vi "printDaqSyncComponent.vi"(8 "error in":errorcluster, 9 "Indent":i32, 10 "TreeRef":refnum<vi>, 11 "baseObject in":refnum<class "IBaseObject.lvclass">) -> (0 "error out":errorcluster, 3 "baseObject out":refnum<class "IBaseObject.lvclass">)   [LabVIEW 2022 SP3, in "openDAQ.lvlib" / "daqUtils.lvlib" / "Tree.lvlib"]
uses:
  Tree.lvlib
  ISyncComponent/ISyncComponent.lvclass
  IBaseObject/IBaseObject.lvclass
  IBaseObject/Polymorphic/queryInterface/querySyncComponentInterface.vi
  IComponent/IComponent.lvclass
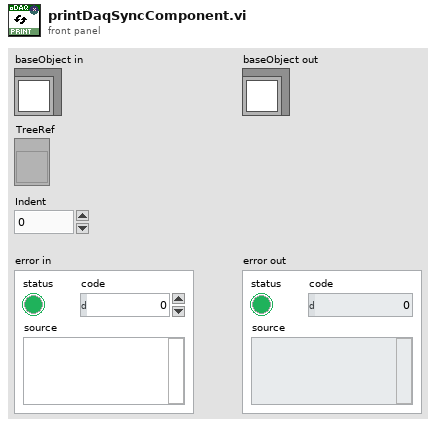
[diagram p1: front panel]
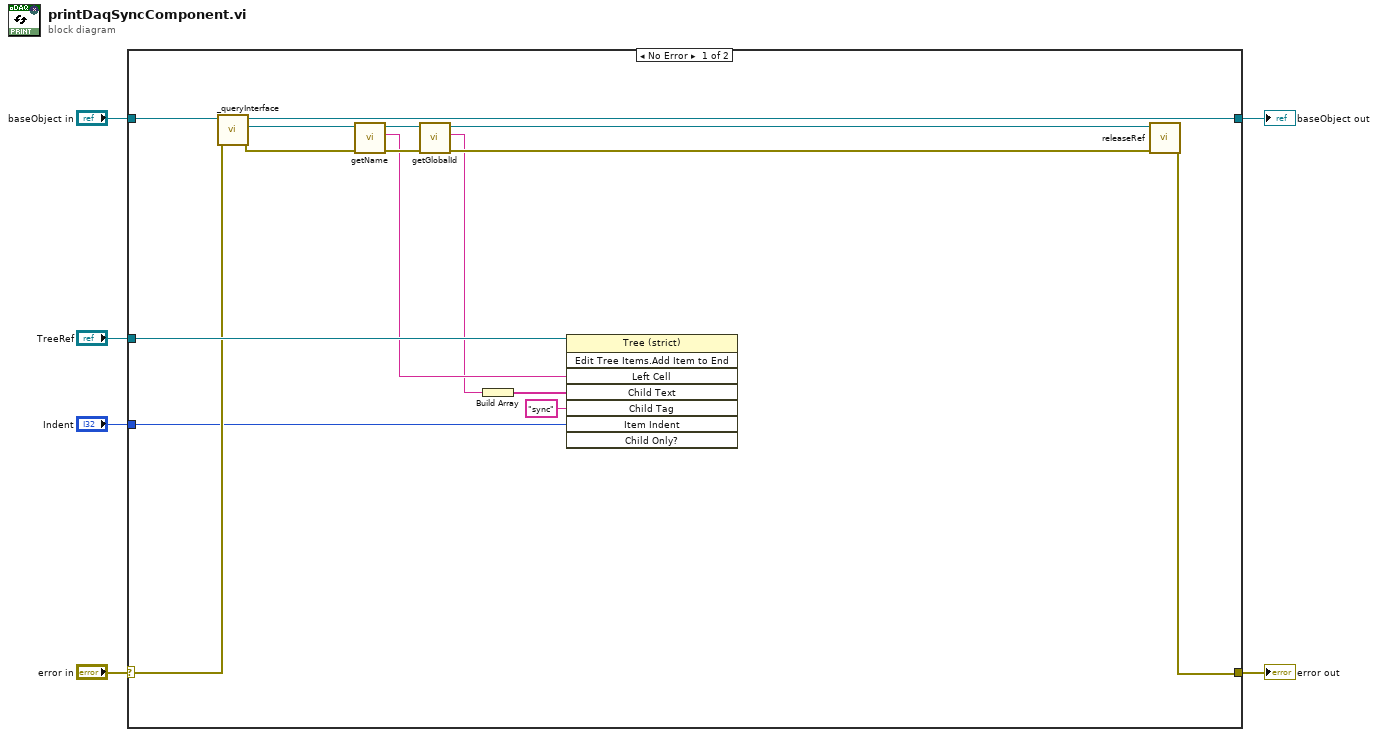
[diagram p0: block diagram]
diagram:
  n1 = case shown="No Error" "error in" {
    selector: "error in" -> [w17 w24]
    tunnel: "baseObject in" -> [w22 w23]
    tunnel: "Indent" -> [w16 _]
    tunnel: "TreeRef" -> [w18 _]
    tunnel: [w15 w24] -> w2
    tunnel: [w20 w23] -> w1
    frame No Error {
      n2 = call-poly "_queryInterface.vi"("error in (no error)"=w17, "IBaseObject in"=w22) -> ("error out"=w19:errorcluster, "ISyncComponent out"=w21:refnum<class "ISyncComponent.lvclass">, "IBaseObject out"=w20:refnum<class "IBaseObject.lvclass">)  [unwired: 7 in]
      n3 = call "getName.vi"("error in (no error)"=w19, "IComponent in"=w21) -> ("error out"=w11:errorcluster, "Name out"=w9:string, "IComponent out"=w13:refnum<class "ISyncComponent.lvclass">)  [unwired: 7 in]
      n4 = call "getGlobalId.vi"("error in (no error)"=w11, "IComponent in"=w13) -> ("error out"=w10:errorcluster, "GlobalId out"=w8:string, "IComponent out"=w12:refnum<class "ISyncComponent.lvclass">)  [unwired: 7 in]
      n5 = Build Array(w8) -> (w7:string[])
      n6 = invoke class="Tree (strict)" method="Edit Tree Items.Add Item to End"(reference=w18, "Left Cell"=w9, "Child Text"=w7, "Child Tag"="sync", "Item Indent"=w16) -> ()  [unwired: 3 in, 8 out]
      n7 = call-dynamic "releaseRef.vi"("error in (no error)"=w10, "IBaseObject in"=w12) -> ("error out"=w15:errorcluster)  [unwired: 9 in]
    }
    frame Error {
    }
  }
  "error out" <- w2
  "baseObject out" <- w1
